vi "logger_api_log_data.vi"(8 "data":variant, 9 "msg":string, 11 "sender":string) -> ()   [LabVIEW 2019]
doc: "Send <b>data</b> to the logger module."
uses:
  common/common data types/common_event_data.ctl
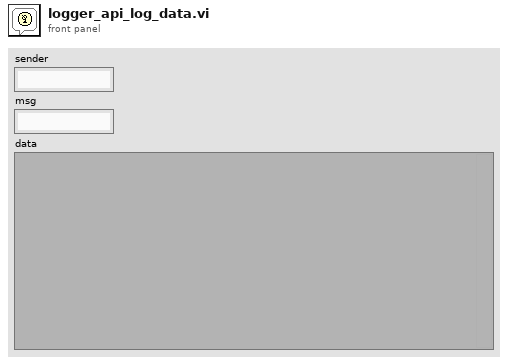
[diagram p1: front panel]
types:
  T1 = typedef "common_event_data.ctl" = cluster{"sender":string, "target":string, "msg":string, "data":variant}
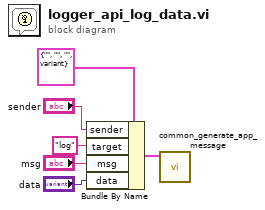
[diagram p0: block diagram]
diagram:
  n1 = Bundle By Name(cluster=T1 {"sender"="", "target"="", "msg"="", "data"=variant} ("event data"), "sender"="sender", "target"="log", "msg"="msg", "data"="data") -> (w6:T1)
  n2 = call "common_generate_app_message.vi"("event data"=w6) -> ()  [unwired: 10 in, 1 out]
